vi "DaqReadFFT.vi"(4 "restart averaging (F)":bool, 5 "dB On":bool=TRUE, 6 "averaging parameters":T2={"averaging mode"=enum."RMS averaging", "weighting mode"=enum."Linear", "number of averages"=100, "linear mode"=enum."One shot"} {"number of averages" min=1 step=1}, 8 "error in":errorcluster caption="错误输入", 9 "channel info":T4={"sensor sensitivity"=1000.0, "engineering units"=3, "dB reference"=2e-05, "custom label"="EU", "weighting filter"=0, "pregain"=0.0} {"pregain" format="%.2f"; "weighting filter" items=["Linear", "A-weighting", "B-weighting", "C-weighting", "ITU-R 468-4", "Dolby", "CCITT", "C-message", "Wb", "Wc", "Wd", "We", "Wf", "Wh", "Wj", "Wk", "Wm", "AES17 20 kHz lowpass", "AES17 40 kHz lowpass", "AES17 20 kHz highpass", "AES17 40 kHz highpass"]; "dB reference" format="%^.1e"; "engineering units" items=["custom..."=0, "V"=1, "A"=21, "C"=30, "pC"=31, "s"=32, "-"=29, "Pa"=2, "N"=20, "g"=3, "m/s^2"=4, "m/s"=5, "m"=6, "mm/s"=12, "mm"=13, "micron/s"=14, "micron"=15, "in/s^2"=7, "in/s"=8, "in"=9, "mil/s"=10, "mil"=11, "rad/s^2"=16, "rad/s"=17, "rad"=18, "deg/s^2"=26, "deg/s"=27, "deg"=28, "RPM"=22, "cycle/s^2"=23, "Hz"=24, "cycle"=25, "strain"=19]; "sensor sensitivity" format="%#_5f"}, 10 "number of samples":i32=2000 min=128, 11 "task out":refnum<k21>) -> (0 "error out":errorcluster, 1 "done":bool, 2 "averages completed":dbl, 3 "task out 2":refnum<k21> caption="任务输出")   [LabVIEW 2018]
uses:
  <vilib>/addons/_NISVFA/_Shared subVIs/Controls/svc_Channel Info.ctl
  <vilib>/addons/_NISVFA/_Shared subVIs/Controls/svc_Engineering Units Text Ring.ctl
  <vilib>/addons/_NISVFA/_Shared subVIs/Controls/svc_Weighting Filter Text Ring.ctl
  <vilib>/addons/_NISVFA/_Shared subVIs/Controls/svc_Window.ctl
  <vilib>/DAQmx/read.llb/DAQmx Read (Analog Wfm 1Chan NSamp).vi
  <vilib>/addons/Sound and Vibration/svt_Calibration/SVL Scale Voltage to EU (1 Ch).vi
  <vilib>/addons/_NISVFA/_Shared subVIs/Common/svc_Set SV Channel Info.vi
  <vilib>/addons/_NISVFA/_Shared subVIs/Common/svc_Set SV Channel Info (variant).vi
  <vilib>/addons/_NISVFA/_Shared subVIs/Common/SVL Set dB Reference (variant).vi
  <vilib>/DAQmx/miscellaneous.llb/DAQmx Fill In Error Info.vi
  <vilib>/addons/_NISVFA/_Shared subVIs/Common/svc_Engineering Units to Unit Label.vi
  <vilib>/addons/_NISVFA/_Shared subVIs/Common/svc_Compute Scale Factor to Convert V to EU.vi
  <vilib>/addons/_NISVFA/_Shared subVIs/Common/svc_Compute Scale Factor to Convert C to EU.vi
  <vilib>/addons/_NISVFA/_Shared subVIs/Common/svc_Set dB ref if Pascal.vi
  <vilib>/addons/_NISVFA/_Shared subVIs/Common/svc_Caller VI Returned in Error Source.vi
  <vilib>/addons/_NISVFA/_Subset FFT/SVFA Power Spectrum Subset (1 Ch).vi
  Global_Variable/A131258.vi
  <vilib>/addons/Sound and Vibration/svt_Calibration/SoundVib_Calibration.lvlib
panel:
  in  "frequency range":T1={"start frequency"=0.0, "stop frequency"=10000.0} {"stop frequency" min=0.0 format="%.2f"; "start frequency" min=0.0 format="%.2f"}
  in  "window":T3=1 items=["None"=0, "Hanning"=1, "Hamming"=2, "Blackman-Harris"=3, "Exact Blackman"=4, "Blackman"=5, "Flat Top"=6, "4 Term B-Harris "=7, "7 Term B-Harris"=8, "Low Sidelobe"=9, "Blackman Nuttall"=11, "Triangle"=30, "Bartlett-Hanning"=31, "Bohman"=32, "Parzen"=33, "Welch"=34, "Kaiser"=60, "Dolph-Chebyshev"=61, "Gaussian"=62]
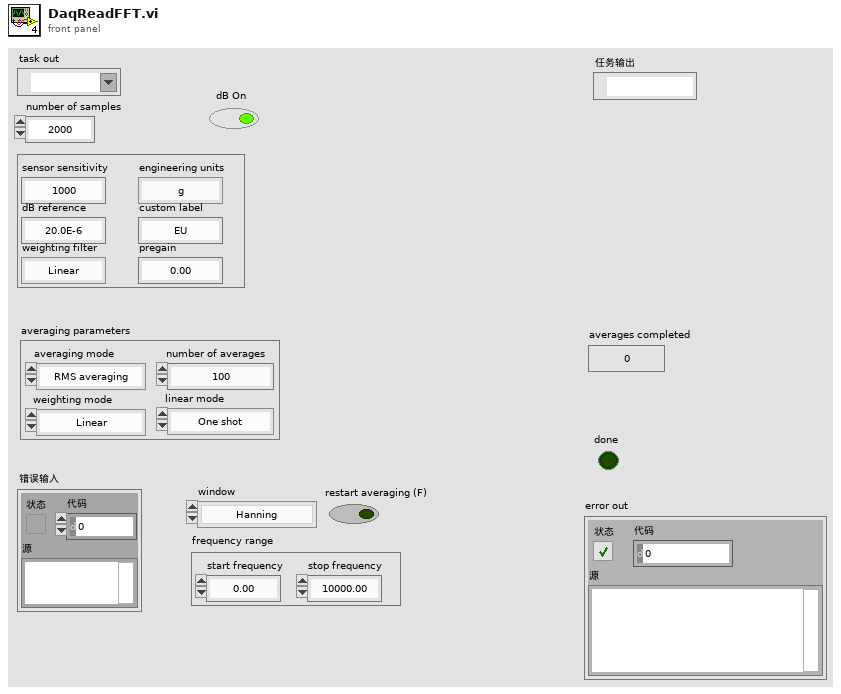
[diagram p1: front panel]
types:
  T1 = cluster{"start frequency":dbl, "stop frequency":dbl}
  T2 = cluster{"averaging mode":enum16{"No averaging", "Vector averaging", "RMS averaging", "Peak hold"}, "weighting mode":enum16{"Linear", "Exponential"}, "number of averages":u32, "linear mode":enum16{"One shot", "Auto restart"}}
  T3 = typedef "svc_Window.ctl" = u32
  T4 = typedef "svc_Channel Info.ctl" = cluster{"sensor sensitivity":dbl, "engineering units":T5, "dB reference":dbl, "custom label":string, "weighting filter":T6, "pregain":dbl}
  T5 = typedef "svc_Engineering Units Text Ring.ctl" = u16
  T6 = typedef "svc_Weighting Filter Text Ring.ctl" = u16
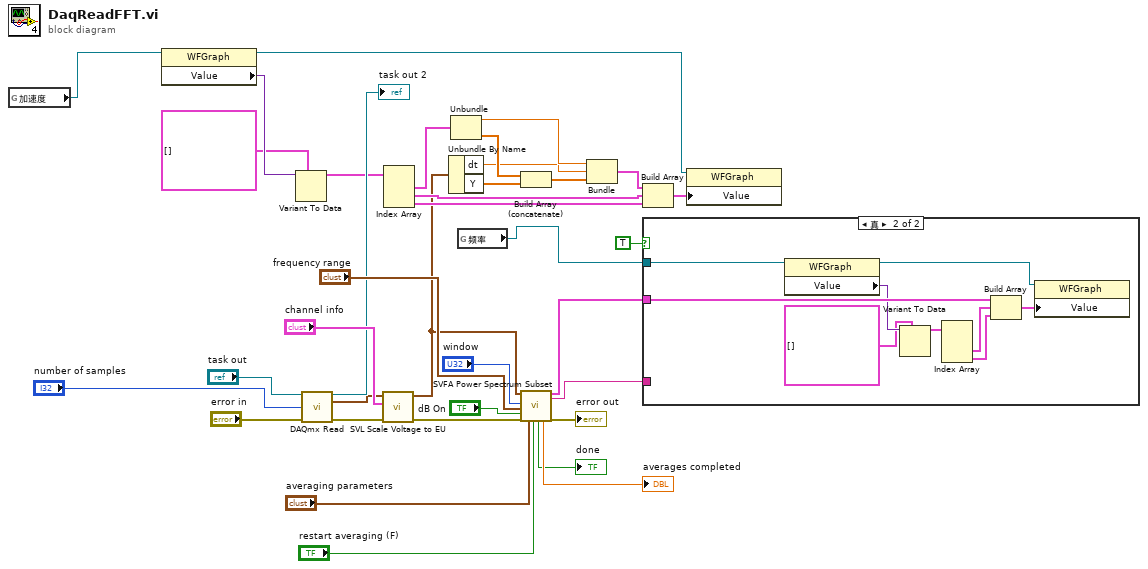
[diagram p0: block diagram]
diagram:
  n1 = global read "A131258.vi" "加速度"() -> (w2:refnum<vi>)
  n2 = property class="WFGraph"(reference=w2) -> (reference out=w17:refnum<vi>, "Value"=w16:variant)  [unwired: 1 in, 1 out]
  n3 = Variant To Data(type=cluster{"f0":dbl, "df":dbl, "magnitude":dbl[]}[] [] ("添加的数组"), Variant=w16) -> (data=w12:cluster{"f0":dbl, "df":dbl, "magnitude":dbl[]}[])  [unwired: 1 in, 1 out]
  n4 = call-poly <vilib>:"DAQmx Read.vi"("task/channels in"="task out", "number of samples per channel"="number of samples", "error in"="error in") -> ("task out"=→"task out 2":refnum<k21>, "data"=w24:waveform(dbl), "error out"=w28:errorcluster)  [unwired: 10 in]
  n5 = call-poly <vilib>:"SVL Scale Voltage to EU.vi"("error in (no error)"=w28, "channel info"="channel info", "signal [V]"=w24) -> ("error out"=w34:errorcluster, "scaled signal [EU]"=w6:waveform(dbl))  [unwired: 6 in, 1 out]
  n6 = Index Array(array=w12) -> (element #1=w7:cluster{"f0":dbl, "df":dbl, "magnitude":dbl[]}, element #2=w10:cluster{"f0":dbl, "df":dbl, "magnitude":dbl[]}, element #3=w11:cluster{"f0":dbl, "df":dbl, "magnitude":dbl[]})  [unwired: 3 in]
  n7 = Unbundle By Name(w6) -> ("dt"=w4:dbl, "Y"=w3:dbl[])
  n8 = Unbundle(w7) -> ("f0"=w15:dbl, "magnitude"=w13:dbl[])  [unwired: 1 out]
  n9 = global read "A131258.vi" "频率"() -> (w1:refnum<vi>)
  n10 = Build Array (concatenate)(w13, w3) -> (w14:dbl[])
  n11 = call-poly <vilib>:"SVFA Power Spectrum Subset.vi"("scaled signal [EU]"=w6, "window"="window", "frequency range"="frequency range", "dB On (T)"="dB On", "error in (no error)"=w34, "averaging parameters"="averaging parameters", "restart averaging (F)"="restart averaging (F)") -> ("averaging done"=→"done":bool, "averages completed"=→"averages completed":dbl, "power spectrum [dB EU]"=w21:cluster{"f0":dbl, "df":dbl, "magnitude":dbl[]}, "unit label"=w20:string, "error out"=→"error out":errorcluster)  [unwired: 7 in, 1 out]
  n12 = Bundle("f0"=w15, "dt"=w4, w14) -> (w9:cluster{"f0":dbl, "dt":dbl, dbl[]})  [unwired: 1 in]
  n13 = Build Array(w9, w10, w11) -> (w8:cluster{"f0":dbl, "df":dbl, "magnitude":dbl[]}[])
  n14 = case shown="真" TRUE ("new spectrum available") {
    tunnel: w21 -> [_ w45]
    tunnel: w20 -> [_ _]
    tunnel: w1 -> [_ w44]
    frame False {
    }
    frame True {
      n15 = property class="WFGraph"(reference=w44) -> (reference out=w42:refnum<vi>, "Value"=w43:variant)  [unwired: 1 in, 1 out]
      n16 = Variant To Data(type=cluster{"f0":dbl, "df":dbl, "magnitude":dbl[]}[] [] ("添加的数组"), Variant=w43) -> (data=w41:cluster{"f0":dbl, "df":dbl, "magnitude":dbl[]}[])  [unwired: 1 in, 1 out]
      n17 = Index Array(array=w41) -> (element #2=w39:cluster{"f0":dbl, "df":dbl, "magnitude":dbl[]}, element #3=w40:cluster{"f0":dbl, "df":dbl, "magnitude":dbl[]})  [unwired: 3 in, 1 out]
      n18 = Build Array(w45, w39, w40) -> (w38:cluster{"f0":dbl, "df":dbl, "magnitude":dbl[]}[])
      n19 = property class="WFGraph"(reference=w42, "Value"=w38) -> ()  [unwired: 1 in, 2 out]
    }
  }
  n20 = property class="WFGraph"(reference=w17, "Value"=w8) -> ()  [unwired: 1 in, 2 out]
